vi "Query WaveIO.vi"() -> (3 "WaveIO Installed":bool)   [LabVIEW 2019, in "Audio Output.lvlib"]
doc: "Checks if the WaveIO DLL is available."
uses:
  Audio Output.lvlib
  external/waveio_108/WaveIO.dll
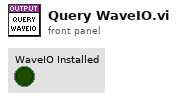
[diagram p1: front panel]
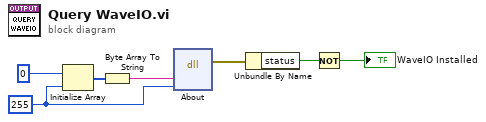
[diagram p0: block diagram]
diagram:
  w5 = 255 ("dimension size")
  n1 = Initialize Array(u8 0 ("element"), w5) -> (w7:u8[])
  n2 = Byte Array To String(unsigned byte array=w7) -> (string=w4:string)
  n3 = dll-call lib="C:/github/dataflowg/dataflow-dj/external/waveio_108/waveio.dll" fn="About"("text"=w4, "txt_size"=w5) -> (error out=w3:errorcluster)  [unwired: 6 in, 1 out]
  n4 = Unbundle By Name(w3) -> ("status"=w2:bool)
  n5 = Not(x=w2) -> (.not. x?=→"WaveIO Installed":bool)
